vi "Burst7.vi"(0 "# bins":refnum<vi>, 1 "binning (s)":refnum<vi>, 3 "% overtalk D-T1":u8, 4 "% overtalk D-T2":u8, 5 "% overtalk D-A":u8, 6 "HydraHarp":bool, 7 "File Number":u32, 8 "channels":u8[](array[numeric]), 9 "x * sigma":u8=3, 12 "MCS":refnum<vi>, 14 "Calculate":bool=TRUE, 15 "Parameters":T1={"PeakThreshold"=30, "RecognitionThreshold"=25, "SeparationLimit"=0.7} {"SeparationLimit" format="%.2f"}, 16 "automatic threshold":bool) -> (13 "mean, std.dev":dbl[](array[numeric]) format="%.2f", 17 "Parameters out":T1, 20 "Intensity Historgram":cluster{"Axis":dbl[], "Histogram":i32[]}(graph), 21 "FRET histogram":cluster{"Axis":dbl[], "Histogram":i32[]}[](graph), 23 "Save F2":dbl[][](array[numeric]) format="%.2f", 24 "Statistik F2":dbl[](array[numeric]) format="%.2f", 27 "# bursts":i32)   [LabVIEW 2009]
uses:
  <vilib>/Utility/file.llb/Write To Spreadsheet File (I64).vi
  <vilib>/Analysis/NI_AALBase.lvlib
  <vilib>/Analysis/NI_AALPro.lvlib
panel:
  in  "Boolean":bool
  out "Histogram Burstwidth / ms":cluster{"Axis":dbl[], "Histogram":i32[]}(graph)
  # "Spot"
  # "burst/s"
  # "bursts"
  # "mean burstwidth / ms"
  # "mean Int"
  # "rec. Thres"
  # "Sum BG"
  # "BG C1"
  # "BGC2"
  # "BG Tr2"
  # "BG Acc"
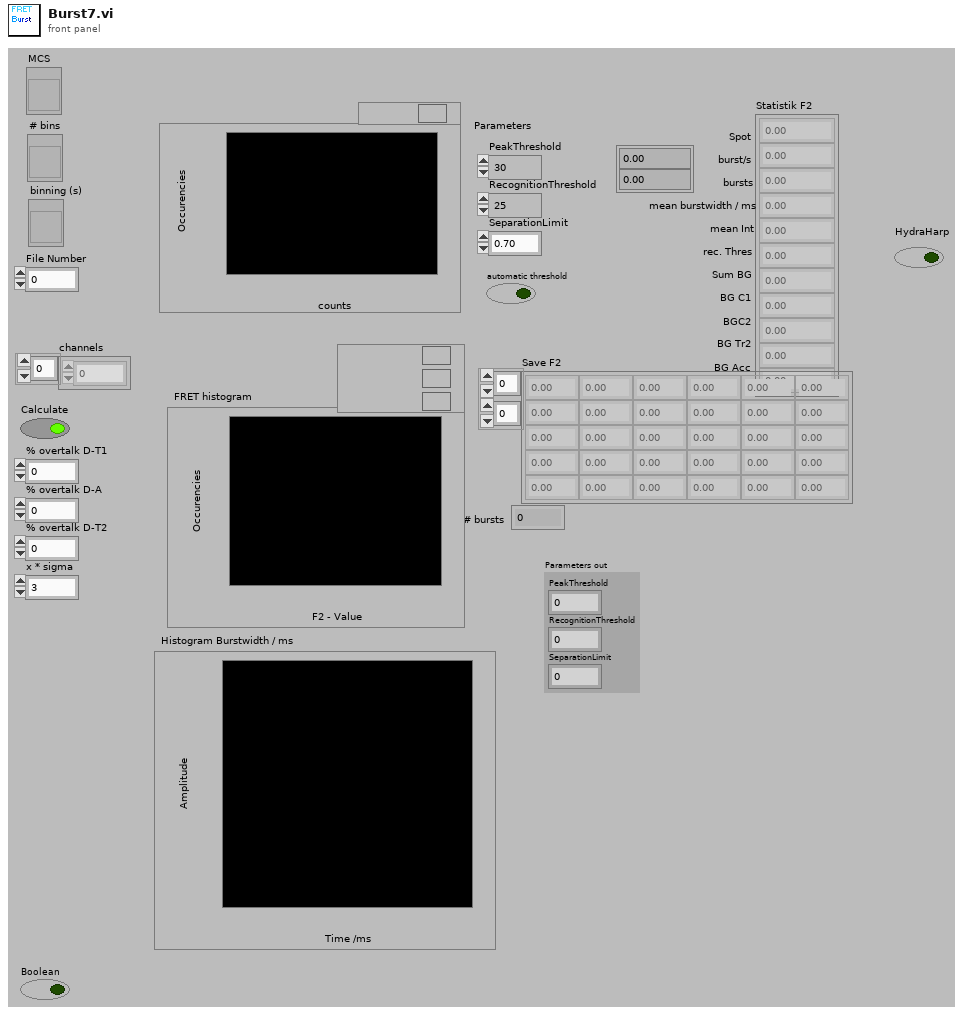
[diagram p1: front panel]
types:
  T1 = cluster{"PeakThreshold":u32, "RecognitionThreshold":u32, "SeparationLimit":sgl}
  T2 = cluster{"router channels":u8[], "macro times":dbl[], "micro times":u16[], "invalid times":u32[], "gap times":u32[]}
  T3 = cluster{"binning (s)":dbl, "binning (s)":dbl, "Histogram: h(x)":u32[]}[]
  T4 = cluster{"binning (s)":dbl, "binning (s)":dbl, "Histogram: h(x)":u32[]}
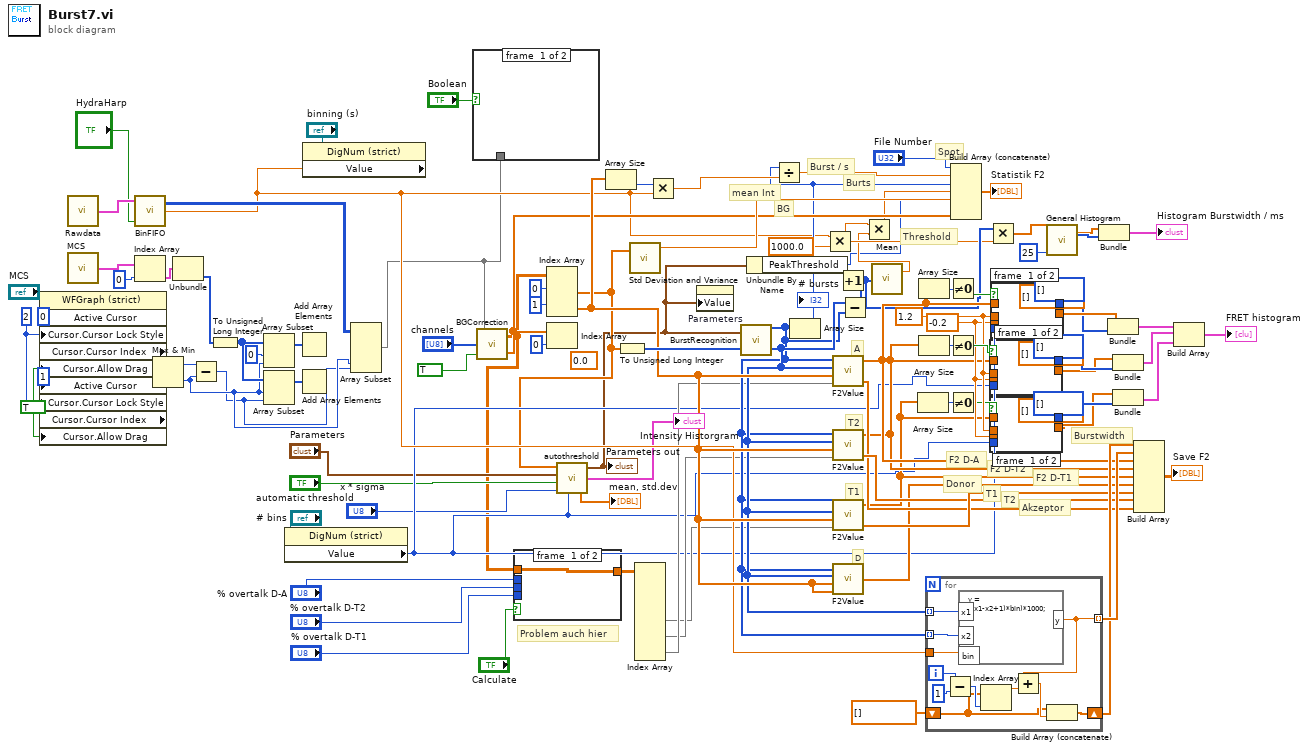
[diagram p0: block diagram]
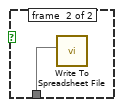
[diagram p2: hidden frame]
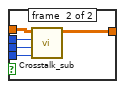
[diagram p3: hidden frame]
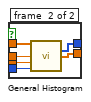
[diagram p4: hidden frame]
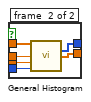
[diagram p5: hidden frame]
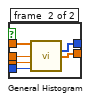
[diagram p6: hidden frame]
diagram:
  (unwired) 0.0 ("x")
  w46 = u32 2 ("Write Attribute")
  w54 = TRUE ("Write Attribute")
  w75 = 1.2 ("min")
  w74 = -0.2 ("max")
  # "Problem auch hier"
  # "D"
  # "T1"
  # "T2"
  # "A"
  # "Akzeptor"
  # "F2 D-T1"
  # "T2"
  # "F2 D-A"
  # "T1"
  # "Donor"
  # "Threshold"
  # "BG"
  # "mean Int"
  # "Burts"
  # "Burst / s"
  # "Spot"
  # "Burstwidth"
  # "F2 D-T2"
  n1 = property on="Property Node" class="WFGraph (strict)"(reference="MCS", "Active Cursor"=u32 0, "Cursor.Cursor Lock Style"=w46, "Cursor.Allow Drag"=w54, "Active Cursor"=u32 1, "Cursor.Cursor Lock Style"=w46, "Cursor.Allow Drag"=w54) -> ("Cursor.Cursor Index"=w53:i32, "Cursor.Cursor Index"=w52:i32)  [unwired: 1 in, 2 out]
  n2 = call "Rawdata.vi"() -> ("output rawdata"=w101:T2)  [unwired: 2 in]
  n3 = call "MCS.vi"() -> ("MCS output"=w41:T3)  [unwired: 2 in]
  n4 = Index Array(array=w41, index=0) -> (element=w56:T4)
  n5 = Max & Min(x=w53, y=w52) -> (max(x,y)=w51:i32, min(x,y)=w39:i32)
  n6 = Unbundle(w56) -> ("Histogram: h(x)"=w47:u32[])  [unwired: 2 out]
  n7 = Subtract(x=w51, y=w39) -> (x-y=w38:i32)
  n8 = To Unsigned Long Integer(number=w47) -> (unsigned 32bit integer=w49:u32[])
  n9 = Array Subset(array=w49, index=0, length=w39) -> (w50:u32[])
  n10 = Array Subset(array=w49, index=w39, length=w38) -> (w55:u32[])
  n11 = property class="DigNum (strict)"(reference="# bins") -> ("Value"=w13:i32)  [unwired: 1 in, 2 out]
  n12 = Add Array Elements(numeric array=w50) -> ()  [unwired: 1 out]
  n13 = Add Array Elements(numeric array=w55) -> ()  [unwired: 1 out]
  n14 = property class="DigNum (strict)"(reference="binning (s)") -> ("Value"=w25:dbl)  [unwired: 1 in, 2 out]
  n15 = call "BinFIFO.vi"("HydraHarp"="HydraHarp", "binning (s)"=w25, "rawdata"=w101) -> ("MCS"=w40:u32[][])  [unwired: 1 out]
  n16 = Array Subset(array=w40, index (col)=w39, length (col)=w38) -> (w3:u32[][])  [unwired: 2 in]
  n17 = case shown="True" "Boolean" {
    tunnel: w3 -> [_ w102]
    frame #0 {
    }
    frame #1 {
      n18 = call-poly <vilib>:"Write To Spreadsheet File.vi"("2D data"=w102) -> ()  [unwired: 7 in, 1 out]
    }
  }
  n19 = call "BGCorrection.vi"("Boolean"=TRUE, "channels"="channels", "MCS"=w3) -> ("BG_mcs"=w58:sgl[], "MCS_bg_corr"=w4:sgl[][])
  n20 = case shown="True" "Calculate" {
    tunnel: "% overtalk D-A" -> [_ w108]
    tunnel: "% overtalk D-T1" -> [_ w107]
    tunnel: "% overtalk D-T2" -> [_ w106]
    tunnel: w4 -> [w103 w104]
    tunnel: [w103 w105] -> w16
    frame #0 {
    }
    frame #1 {
      n21 = call "Crosstalk_sub.vi"("% overtalk D-T1"=w107, "% overtalk D-T2"=w106, "% overtalk D-A"=w108, "MCS_bg_corr"=w104) -> ("MCS_crosstalk_corr"=w105:dbl[][])  [unwired: 3 out]
    }
  }
  n22 = Index Array(array=w4, index (row) #1=0 ("index"), index (row) #2=1 ("index (row)")) -> (element #1=w12:sgl[], element #2=w59:sgl[])  [unwired: 2 in]
  n23 = Index Array(array=w58, index=0) -> ()  [unwired: 1 out]
  n24 = call "autothreshold.vi"("MCS_bg_corr"=w12, "Parameters in"="Parameters", "automatic threshold"="automatic threshold", "x * sigma"="x * sigma", "# bins"=w13) -> ("Parameters out"=w6:T1, "Intensity Historgram"=→"Intensity Historgram":cluster{"Axis":dbl[], "Histogram":i32[]}, "mean, std.dev"=→"mean, std.dev":dbl[])
  "Parameters out" <- w6
  n25 = Array Size(array=w59) -> (size(s)=w98:i32)
  n26 = To Unsigned Long Integer(number=w12) -> (unsigned 32bit integer=w83:u32[])
  n27 = call "Std Deviation and Variance.vi"("X"=w12) -> ("mean"=w96:dbl)  [unwired: 1 in, 2 out]
  n28 = Index Array(array=w16) -> (element #3=w17:dbl[], element #4=w18:dbl[], element #5=w19:dbl[])  [unwired: 10 in, 2 out]
  n29 = Multiply(x=w98, y=w25) -> (x*y=w37:dbl)
  n30 = property on="Parameters" class="Cluster (strict)"("Value"=w6) -> ()  [unwired: 2 in, 2 out]
  n31 = call "BurstRecognition.vi"("IntensityTrace"=w83, "Parameters"=w6) -> ("Index Hi"=w35:u32[], "Index Low"=w34:u32[])
  n32 = Unbundle By Name(w6) -> ("PeakThreshold"=w5:u32)
  n33 = Array Size(array=w34) -> (size(s)=w36:i32)
  "# bursts" <- w36
  n34 = Divide(x=w36, y=w37) -> (x/y=w97:dbl)
  n35 = Multiply(x=w25, y=1000.0) -> (x*y=w24:dbl)
  n36 = call "F2Value.vi"("channel 2"=w19, "channel1"=w59, "Index Hi"=w35, "Index Low"=w34) -> ("channel2 out"=w84:dbl[], "F2-values"=w80:dbl[])  [unwired: 1 out]
  n37 = call "F2Value.vi"("channel 2"=w18, "channel1"=w59, "Index Hi"=w35, "Index Low"=w34) -> ("channel2 out"=w85:dbl[], "F2-values"=w65:dbl[])  [unwired: 1 out]
  n38 = call "F2Value.vi"("channel 2"=w17, "channel1"=w59, "Index Hi"=w35, "Index Low"=w34) -> ("channel2 out"=w86:dbl[], "F2-values"=w64:dbl[])  [unwired: 1 out]
  n39 = call "F2Value.vi"("channel 2"=w59, "channel1"=w59, "Index Hi"=w35, "Index Low"=w34) -> ("channel1 out"=w82:dbl[])  [unwired: 2 out]
  n40 = Subtract(x=w35, y=w34) -> (x-y=w28:u32[])
  n41 = Increment(x=w28) -> (x+1=w27:u32[])
  n42 = call <vilib>:"Mean.vi"("X"=w27) -> ("mean"=w23:dbl)  [unwired: 1 out]
  n43 = Multiply(x=w24, y=w23) -> (x*y=w33:dbl)
  n44 = Array Size(array=w64) -> (size(s)=w73:i32)
  n45 = Array Size(array=w80) -> (size(s)=w26:i32)
  n46 = Array Size(array=w65) -> (size(s)=w77:i32)
  n47 = for {
    tunnel: w35 -> [w119] mode=indexing
    tunnel: w34 -> [w118] mode=indexing
    tunnel: [w113] -> w92 mode=indexing
    tunnel: w25 -> [w117]
    shift-right: [w111] -> w90
    shift-left: dbl[] [] -> [w110]
    i -> [w116]
    n48 = Subtract(x=w116, y=1) -> (x-y=w114:i32)
    n49 = formula code="y = ((x1-x2+1)*bin)*1000;"("x1"=w119, "x2"=w118, "bin"=w117) -> ("y"=w113:dbl)
    n50 = Index Array(array=w110, index=w114) -> (element=w109:dbl)
    n51 = Add(x=w113, y=w109) -> (x+y=w112:dbl)
    n52 = Build Array (concatenate)(w110, w112) -> (w111:dbl[])
  }
  n53 = Not Equal To 0?(x=w26) -> (x != 0?=w81:bool)
  n54 = Not Equal To 0?(x=w77) -> (x != 0?=w76:bool)
  n55 = Not Equal To 0?(x=w73) -> (x != 0?=w72:bool)
  n56 = Build Array (concatenate)("File Number", w97, w36, w33, w96, w5, w58) -> (→"Statistik F2":dbl[])
  n57 = Multiply(x=w27, y=w24) -> (x*y=w21:dbl[])
  n58 = case shown="True" w76 {
    tunnel: w65 -> [_ w127]
    tunnel: [i32[] [] ("Histogram") w126] -> w71
    tunnel: [dbl[] [] ("Axis") w125] -> w70
    tunnel: w74 -> [_ w124]
    tunnel: w75 -> [_ w123]
    tunnel: w13 -> [_ w122]
    frame #0 {
    }
    frame #1 {
      n59 = call <vilib>:"General Histogram.vi"("X"=w127, "max"=w123, "min"=w124, "# bins"=w122) -> ("Histogram"=w126:i32[], "Axis"=w125:dbl[])  [unwired: 7 in, 3 out]
    }
  }
  n60 = case shown="True" w72 {
    tunnel: w64 -> [_ w135]
    tunnel: [i32[] [] ("Histogram") w134] -> w67
    tunnel: [dbl[] [] ("Axis") w133] -> w66
    tunnel: w74 -> [_ w132]
    tunnel: w75 -> [_ w131]
    tunnel: w13 -> [_ w130]
    frame #0 {
    }
    frame #1 {
      n61 = call <vilib>:"General Histogram.vi"("X"=w135, "max"=w131, "min"=w132, "# bins"=w130) -> ("Histogram"=w134:i32[], "Axis"=w133:dbl[])  [unwired: 7 in, 3 out]
    }
  }
  n62 = case shown="True" w81 {
    tunnel: w80 -> [_ w143]
    tunnel: [i32[] [] ("Histogram") w142] -> w78
    tunnel: [dbl[] [] ("Axis") w141] -> w79
    tunnel: w74 -> [_ w140]
    tunnel: w75 -> [_ w139]
    tunnel: w13 -> [_ w138]
    frame #0 {
    }
    frame #1 {
      n63 = call <vilib>:"General Histogram.vi"("X"=w143, "max"=w139, "min"=w140, "# bins"=w138) -> ("Histogram"=w142:i32[], "Axis"=w141:dbl[])  [unwired: 7 in, 3 out]
    }
  }
  n64 = call <vilib>:"General Histogram.vi"("X"=w21, "# bins"=25) -> ("Histogram"=w32:i32[], "Axis"=w31:dbl[])  [unwired: 9 in, 3 out]
  n65 = Bundle("Axis"=w31, "Histogram"=w32) -> (→"Histogram Burstwidth / ms":cluster{"Axis":dbl[], "Histogram":i32[]})  [unwired: 1 in]
  n66 = Bundle("Axis"=w79, "Histogram"=w78) -> (w89:cluster{"Axis":dbl[], "Histogram":i32[]})  [unwired: 1 in]
  n67 = Bundle("Axis"=w70, "Histogram"=w71) -> (w69:cluster{"Axis":dbl[], "Histogram":i32[]})  [unwired: 1 in]
  n68 = Bundle("Axis"=w66, "Histogram"=w67) -> (w68:cluster{"Axis":dbl[], "Histogram":i32[]})  [unwired: 1 in]
  n69 = Build Array(w90, w92, w80, w65, w64, w82, w86, w85, w84) -> (→"Save F2":dbl[][])
  n70 = Build Array(w89, w69, w68) -> (→"FRET histogram":cluster{"Axis":dbl[], "Histogram":i32[]}[])
